vi "FaKI State Machine.vi"() -> ()   [LabVIEW 2023, in "FaKI State Machine.lvlib"]
doc: "The Producer-Consumer version of JKI State Machine.\n\nThis VI template must be instantiated by placing it on the block diagram of a new blank VI directly from the palettes. Do not use this template directly."
uses:
  FaKI State Machine.lvlib
  <vilib>/Utility/error.llb/Clear Errors.vi
panel:
  in  "Exit":bool
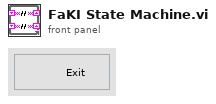
[diagram p1: front panel]
types:
  T1 = enum32{"Invalid", "Standard", "Closed", "Hidden", "Minimized", "Maximized"}
  T2 = enum32{"invalid app kind", "Development System", "Run Time System", "Student Edition", "Embedded LabVIEW", "Evaluation", "Custom"}
  T3 = cluster{"Core":cluster{"Current VI Reference":refnum<vi>, "Close Panel on Exit?":bool}, "Your Boolean data":bool, "Your string data":string}
  T4 = cluster{"Current VI Reference":refnum<vi>, "Close Panel on Exit?":bool}
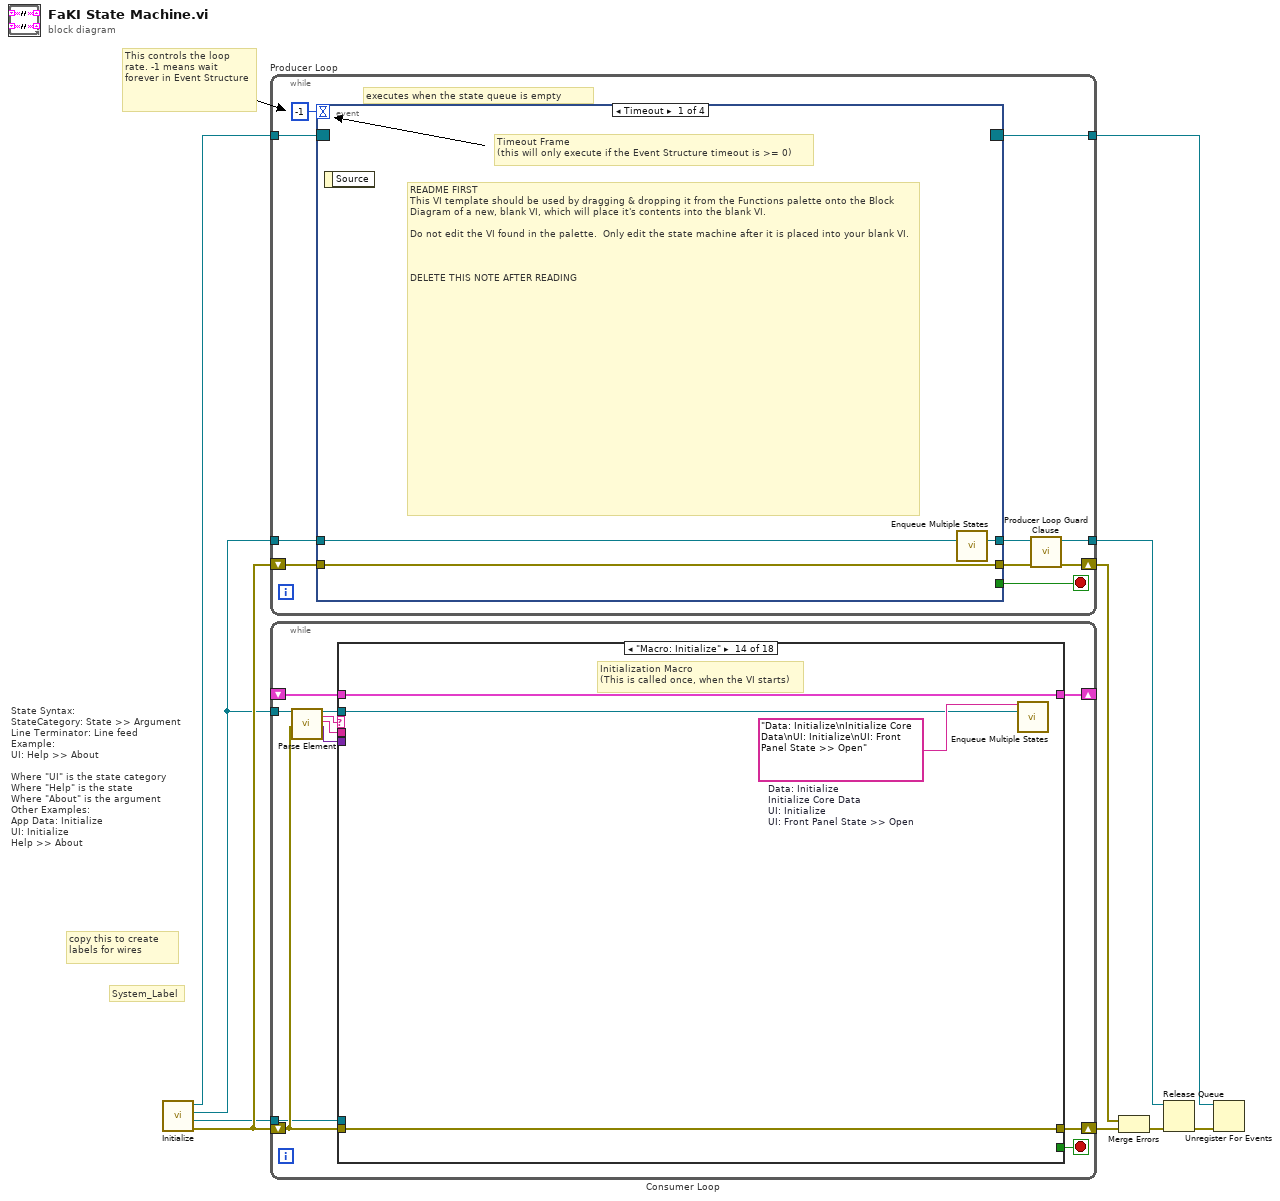
[diagram p0: block diagram]
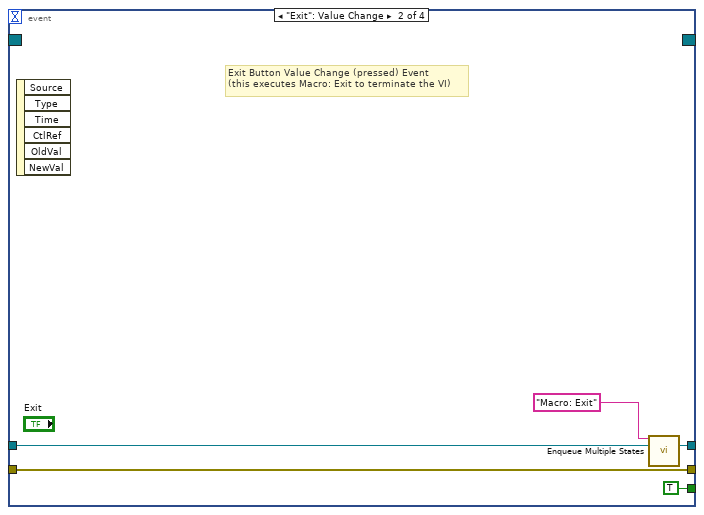
[diagram p2: hidden frame]
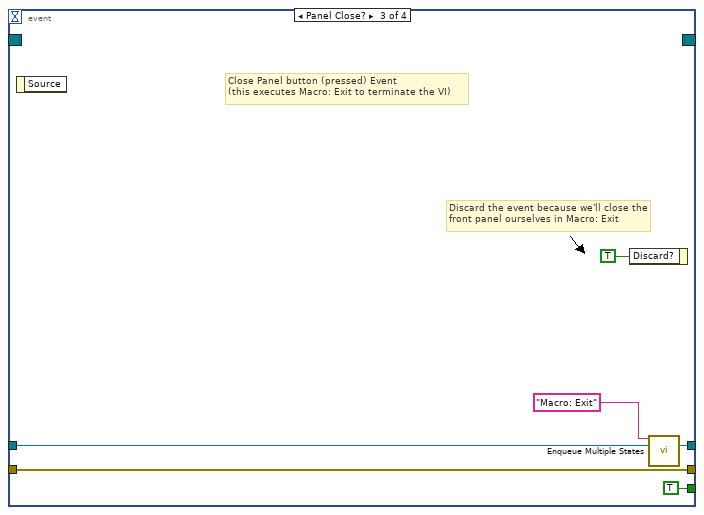
[diagram p3: hidden frame]
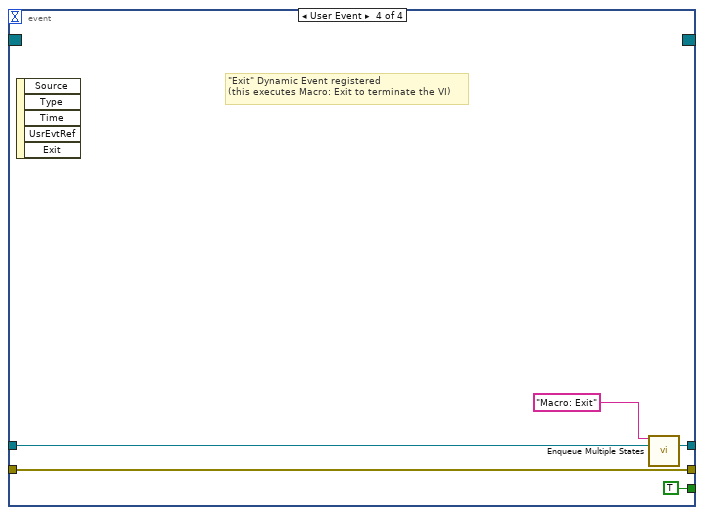
[diagram p4: hidden frame]
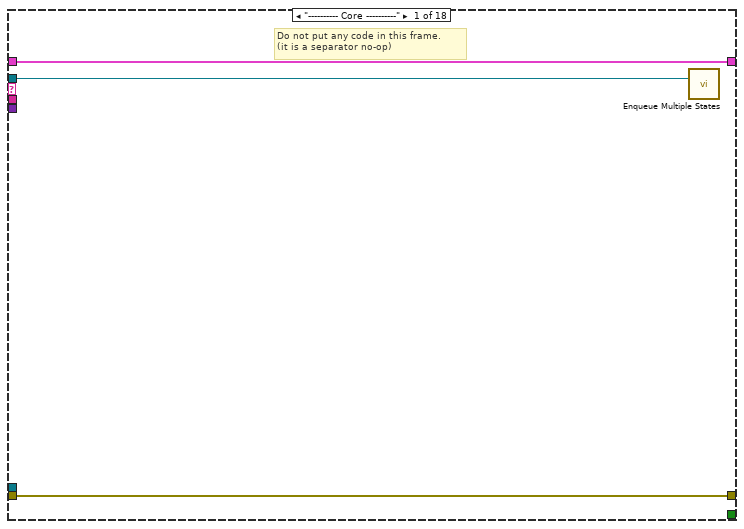
[diagram p5: hidden frame]
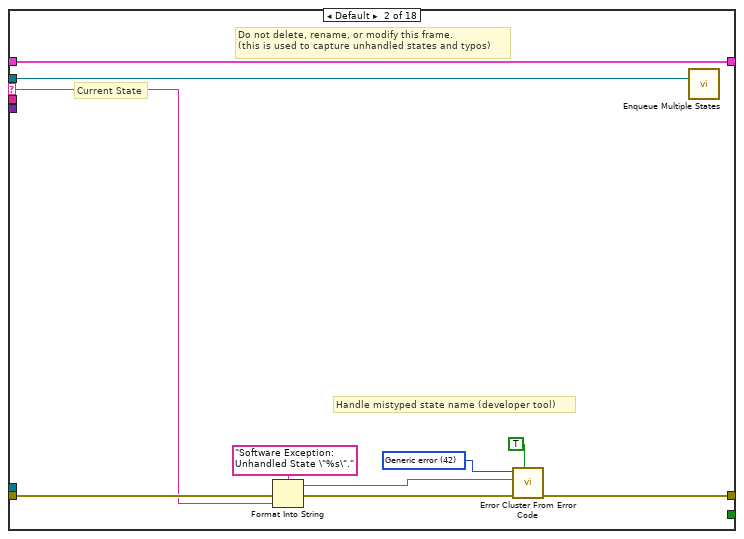
[diagram p6: hidden frame]
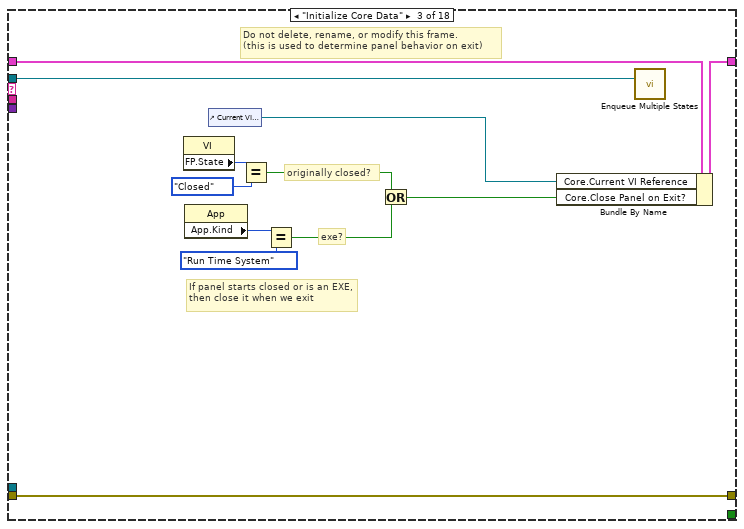
[diagram p7: hidden frame]
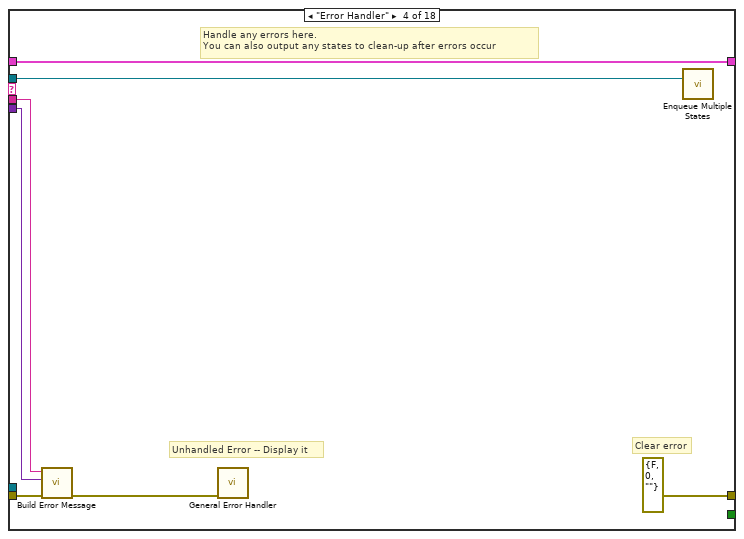
[diagram p8: hidden frame]
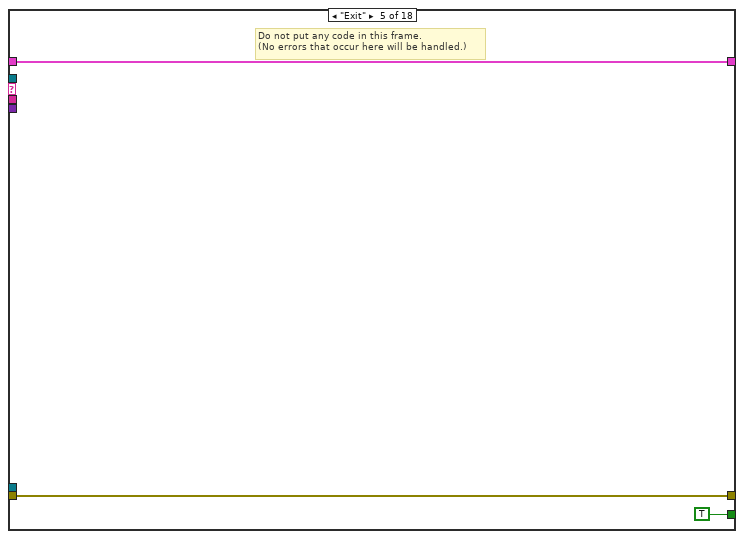
[diagram p9: hidden frame]
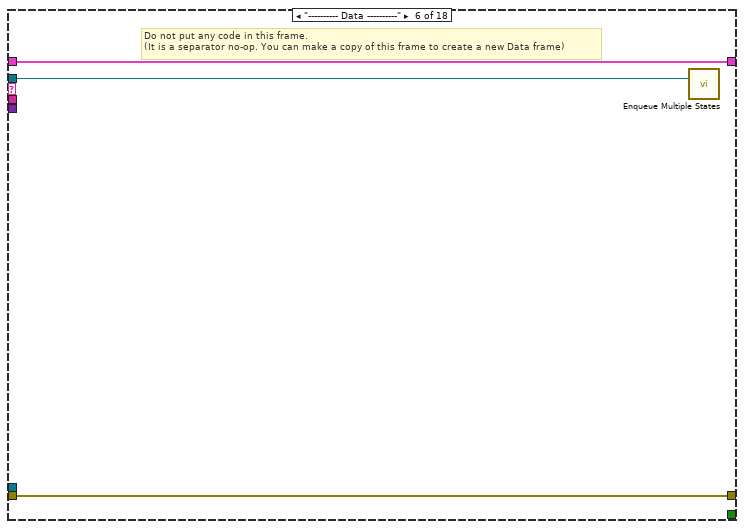
[diagram p10: hidden frame]
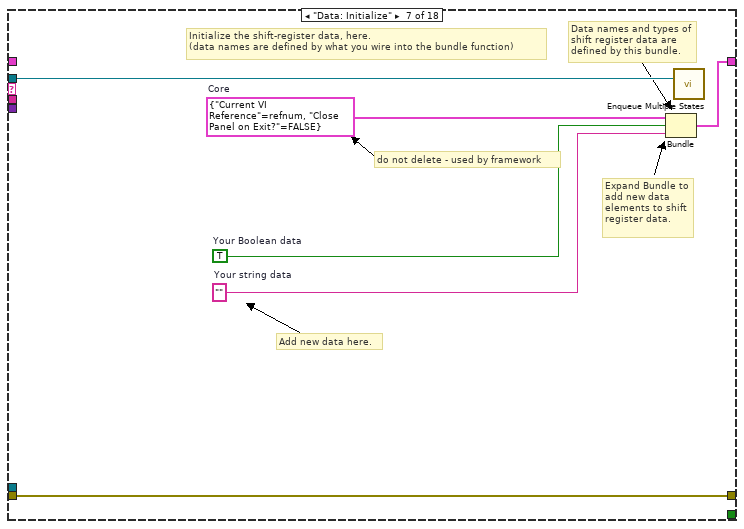
[diagram p11: hidden frame]
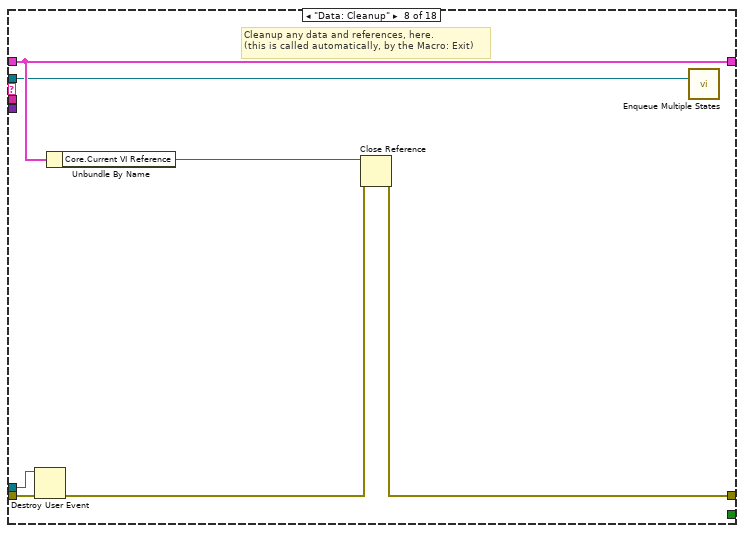
[diagram p12: hidden frame]
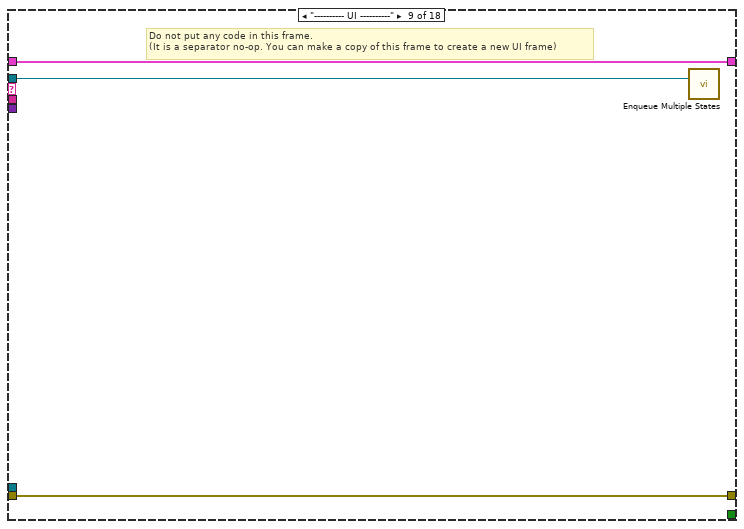
[diagram p13: hidden frame]
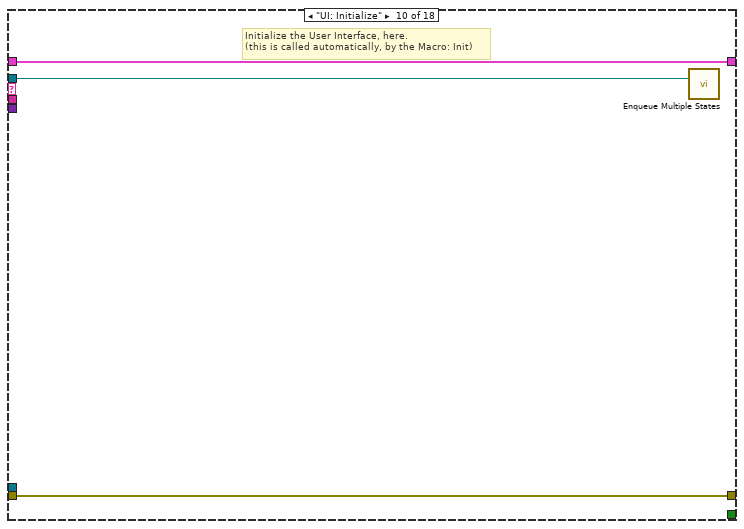
[diagram p14: hidden frame]
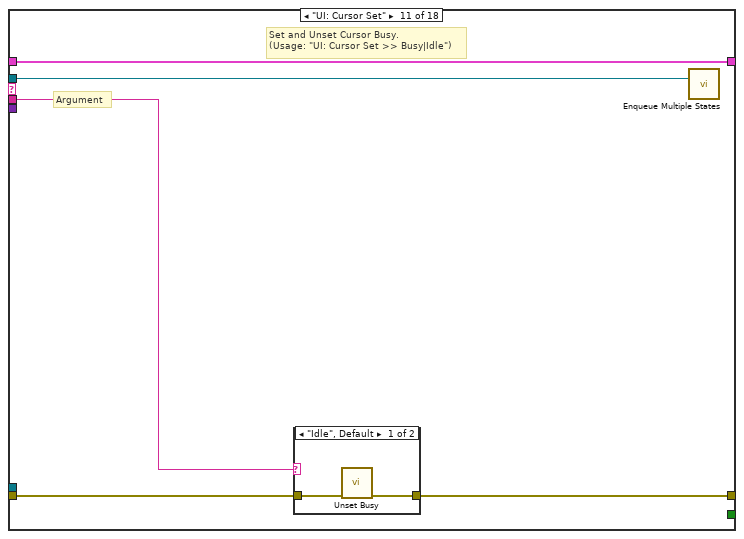
[diagram p15: hidden frame]
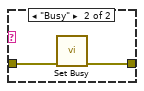
[diagram p16: hidden frame]
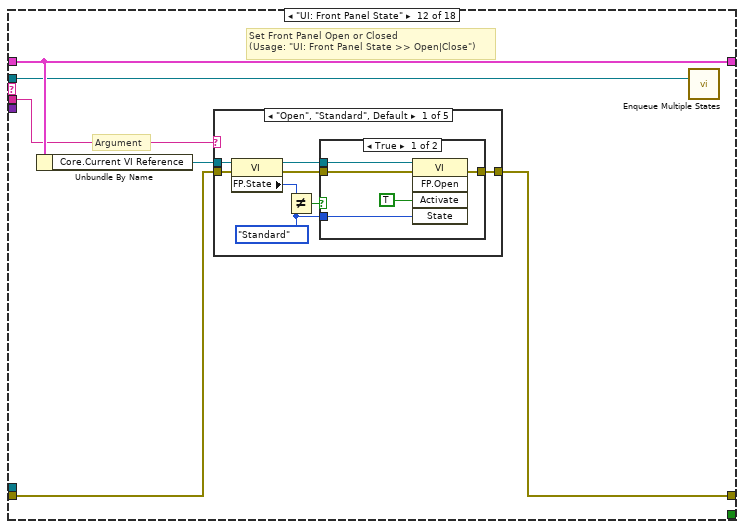
[diagram p17: hidden frame]
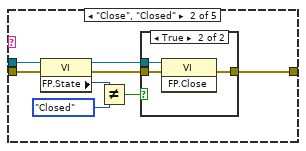
[diagram p19: hidden frame]
diagram:
  # "This controls the loop rate. -1 means wait forever in Event Structure"
  # "State Syntax:\nStateCategory: State >> Argument\nLine Terminator: Line feed\nExample:\nUI: Help >> About\n\nWhere \"UI\" is the state category\nWhere \"Help\" is the state\nWhere \"About\" is the argument\nOther Examples:\nApp Data: Initialize\nUI: Initialize\nHelp >> About"
  # "copy this to create labels for wires"
  # "System_Label"
  n1 = call "Initialize.vi"() -> ("error out"=w6:errorcluster, "Exit Event out"=w3:refnum<user-event>, "queue out"=w5:refnum<queue>, "Event Registration Refnum out"=w4:refnum<event-registration>)  [unwired: 8 in]
  n2 = while "Producer Loop" {
    shift-right: [w15] -> w9
    shift-left: w6 -> [w20]
    tunnel: w4 -> [w12]
    tunnel: w5 -> [w18]
    tunnel: [w13] -> w7
    tunnel: [w11] -> w1
    stop <- w17 stop-if-true
    # "executes when the state queue is empty"
    n3 = event shown="[0] Timeout" {
      selector: w12 -> [_ _ _ _]
      dyn-events: [_ _ _ _] -> w11
      timeout: -1 ("Timeout") -> [_ _ _ _]
      tunnel: [w21 w28 w34 w39] -> w16
      tunnel: w20 -> [w21 w28 w34 w39]
      tunnel: w18 -> [w22 w27 w31 w37]
      tunnel: [w23 w25 w30 w36] -> w14
      tunnel: [_ TRUE TRUE TRUE] -> w17
      event Timeout {
        # "README FIRST\nThis VI template should be used by dragging & dropping it from the Functions palette onto the Block Diagram of a new, blank VI, which will place it's contents into the blank VI.\n\nDo not edit the VI found in the palette.  Only edit the state machine after it is placed into your blank VI.\n\n\n\nDELETE THIS NOTE AFTER READING"
        # "Timeout Frame\n(this will only execute if the Event Structure timeout is >= 0)"
        n4 = event-data() -> ()  [unwired: 1 in, 1 out]
        n5 = call "Enqueue Multiple States.vi"("queue in"=w22) -> ("queue out"=w23:refnum<queue>)  [unwired: 14 in]
      }
      event "Exit": Value Change {
        # "Exit Button Value Change (pressed) Event\n(this executes Macro: Exit to terminate the VI)"
        n6 = event-data() -> ()  [unwired: 1 in, 6 out]
        n7 = call "Enqueue Multiple States.vi"("State(s) at Front"="Macro: Exit", "queue in"=w27) -> ("queue out"=w25:refnum<queue>)  [unwired: 13 in]
      }
      event Panel Close? {
        # "Discard the event because we'll close the front panel ourselves in Macro: Exit"
        # "Close Panel button (pressed) Event\n(this executes Macro: Exit to terminate the VI)"
        n8 = event-data() -> ()  [unwired: 1 in, 1 out]
        n9 = event-data("Discard?"=TRUE) -> ()  [unwired: 1 in, 1 out]
        n10 = call "Enqueue Multiple States.vi"("State(s) at Front"="Macro: Exit", "queue in"=w31) -> ("queue out"=w30:refnum<queue>)  [unwired: 13 in]
      }
      event User Event {
        # "\"Exit\" Dynamic Event registered\n(this executes Macro: Exit to terminate the VI)"
        n11 = event-data() -> ()  [unwired: 1 in, 5 out]
        n12 = call "Enqueue Multiple States.vi"("State(s) at Front"="Macro: Exit", "queue in"=w37) -> ("queue out"=w36:refnum<queue>)  [unwired: 13 in]
      }
    }
    n13 = call "Producer Loop Guard Clause.vi"("error in (no error)"=w16, "queue in"=w14) -> ("error out"=w15:errorcluster, "queue out"=w13:refnum<queue>)  [unwired: 8 in]
  }
  n14 = while "Consumer Loop" {
    shift-right: [w47] -> _
    shift-left: _ -> [w46]
    shift-right: [w50] -> w10
    shift-left: w6 -> [w49]
    tunnel: w5 -> [w45]
    tunnel: w3 -> [w40]
    stop <- w48 stop-if-true
    n15 = call "Parse Element.vi"("queue in"=w45, "error in (no error)"=w49) -> ("queue out"=w44:refnum<queue>, "State"=w43:string, "Arg"=w42:string, "Data"=w41:variant)  [unwired: 14 in]
    n16 = case shown="\"Macro: Initialize\"" w43 {
      selector: w43 -> [_ w55 _ _ _ _ _ _ _ _ _ _ _ _ _ _ _ _]
      tunnel: w44 -> [w51 w54 w64 w80 _ w86 w89 w98 w102 w105 w108 w117 w188 w191 w198 w204 w207 w210]
      tunnel: w42 -> [_ _ _ w76 _ _ _ _ _ _ w109 w118 _ _ _ _ _ _]
      tunnel: w46 -> [w52 w57 w70 w81 w84 w87 _ w99 w103 w106 w110 w120 w189 w193 w202 w205 w208 w211]
      tunnel: [w53 w62 w75 errorcluster {"status"=FALSE, "code"=0, "source"=""} ("error out") w85 w88 w94 w101 w104 w107 w111 w121 w190 w194 w203 w206 w209 w212] -> w50
      tunnel: w49 -> [w53 w61 w75 w79 w85 w88 w94 w97 w104 w107 w112 w122 w190 w194 w203 w206 w209 w212]
      tunnel: [_ _ _ _ TRUE _ _ _ _ _ _ _ _ _ _ _ _ _] -> w48
      tunnel: [w52 w57 w74 w81 w84 w87 w93 w99 w103 w106 w110 w120 w189 w193 w202 w205 w208 w211] -> w47
      tunnel: w41 -> [_ _ _ w77 _ _ _ _ _ _ _ _ _ _ _ _ _ _]
      tunnel: w40 -> [_ _ _ _ _ _ _ w96 _ _ _ _ _ _ _ _ _ _]
      frame "---------- Core ----------" {
        # "Do not put any code in this frame.\n(it is a separator no-op)"
        n17 = call "Enqueue Multiple States.vi"("queue in"=w51) -> ()  [unwired: 14 in, 1 out]
      }
      frame Default {
        w59 = 42 items=["No error", "Argument error", "Memory is full", "Out of zone", "End of file", "File already open", "Generic file I/O error", "File not found", "File permission error", "Disk is full", "Duplicate path", "Too many files open", "System feature not enabled", "Resource file not found", "Cannot add resource", "Resource not found", "Image not found", "Image memory error", "Pen does not exist", "Config type invalid", "Config token not found", "Config parse error", "Config memory error", "Bad external code format", "Bad external code offset", "External code not present", "Null window", "Destroy window error", "Null menu", "Print aborted", "Bad print record", "Print driver error", "Windows error during printing", "Memory error during printing", "Print dialog error", "Generic print error", "Invalid device refnum", "Device not found", "Device parameter error", "Device unit error", "Cannot open device", "Device call aborted", "Generic error", "Cancelled by user", "Object ID too low", "Object ID too high", "Object not in heap", "Unknown heap", "Unknown object (invalid DefProc)", "Unknown object (DefProc not in table)", "Message out of range", "Invalid (null) method", "Unknown message", "Manager call not supported", "Bad address", "Network operation in progress", "Network operation timed out", "Connection is busy", "Network attribute not supported", "Network error", "Address in use", "System out of memory", "Connection aborted", "Connection refused", "Not connected", "Already connected", "Connection closed", "Initialization error (interapplication manager)", "Bad occurrence", "Wait on unbound occurrence handler", "Occurrence queue overflow", "Datalog type conflict", "Unused", "Unrecognized type (interapplication manager)", "Memory corrupt", "Failed to make temporary DLL", "Old CIN version", "Drag socket not found", "Failed to load drop-object", "Failed to register OLE object", "Failed to release OLE object", "Format specifier type mismatch", "Unknown format specifier", "Too few format specifiers", "Too many format specifiers", "Scan failed", "Newer CIN version", "Error converting to variant", "Runtime menu error", "Password tampered", "Variant attribute not found", "Incompatible variant data type", "Event data is not available", "Event Store is not present", "Occurrence is not found", "Event Queue is not created", "Event info is not available", "Refnum passed is NULL", "Error retrieving Class GUID", "Error retrieving CoClass GUID", "Error retrieving TypeLib GUID.", "Bad built application magic bytes.", "Specific driver is different from the specific driver associated with the Logical Name.", "There is no session opened to the class driver.", "Max Error", "MAX - Error with config objects", "MAX - Error loading configuration", "MAX - Group not supported"]
        # "Current State"
        # "Do not delete, rename, or modify this frame.\n(this is used to capture unhandled states and typos)"
        # "Handle mistyped state name (developer tool)"
        n18 = Format Into String(format string="Software Exception: Unhandled State \"%s\"." ("message"), error in=w61, w55) -> (resulting string=w58:string, error out=w63:errorcluster)  [unwired: 1 in]
        n19 = call <vilib>:"Error Cluster From Error Code.vi"("show call chain? (False)"=TRUE, "error in (no error)"=w63, "error message (\"\")"=w58, "error code (0)"=w59) -> ("error out"=w62:errorcluster)  [unwired: 5 in]
        n20 = call "Enqueue Multiple States.vi"("queue in"=w54) -> ()  [unwired: 14 in, 1 out]
      }
      frame "Initialize Core Data" {
        # "Do not delete, rename, or modify this frame.\n(this is used to determine panel behavior on exit)"
        # "originally closed?"
        # "exe?"
        # "If panel starts closed or is an EXE, then close it when we exit"
        n21 = property class="VI"() -> ("FP.State"=w67:T1)  [unwired: 2 in, 2 out]
        n22 = property class="App"() -> ("App.Kind"=w73:T2)  [unwired: 2 in, 2 out]
        n23 = control-ref of="Current VI Reference"() -> (w68:refnum<vi>)
        n24 = Equal?(x=w67, y=T1."Closed" ("Front Panel Window:State")) -> (x = y?=w65:bool)
        n25 = Equal?(x=w73, y=T2."Run Time System" ("Application:Kind")) -> (x = y?=w71:bool)
        n26 = Or(x=w65, y=w71) -> (x .or. y?=w69:bool)
        n27 = Bundle By Name(cluster=w70, "Core.Current VI Reference"=w68, "Core.Close Panel on Exit?"=w69) -> (w74:T3)
        n28 = call "Enqueue Multiple States.vi"("queue in"=w64) -> ()  [unwired: 14 in, 1 out]
      }
      frame "Error Handler" {
        # "Unhandled Error -- Display it"
        # "Handle any errors here.\nYou can also output any states to clean-up after errors occur"
        # "Clear error"
        n29 = call "Build Error Message.vi"("error in (no error)"=w79, "Data"=w77, "Arg"=w76) -> ("error out"=w78:errorcluster)  [unwired: 8 in]
        n30 = call <vilib>:"General Error Handler.vi"("error in (no error)"=w78) -> ()  [unwired: 10 in, 5 out]
        n31 = call "Enqueue Multiple States.vi"("queue in"=w80) -> ()  [unwired: 14 in, 1 out]
      }
      frame "Exit" {
        # "Do not put any code in this frame.\n(No errors that occur here will be handled.)"
      }
      frame "---------- Data ----------" {
        # "Do not put any code in this frame.\n(It is a separator no-op. You can make a copy of this frame to create a new Data frame)"
        n32 = call "Enqueue Multiple States.vi"("queue in"=w86) -> ()  [unwired: 14 in, 1 out]
      }
      frame "Data: Initialize" {
        w90 = T4 {"Current VI Reference"=refnum, "Close Panel on Exit?"=FALSE}  # Core
        w92 = TRUE  # Your Boolean data
        w91 = ""  # Your string data
        # "do not delete - used by framework"
        # "Expand Bundle to add new data elements to shift register data."
        # "Add new data here."
        # "Data names and types of shift register data are defined by this bundle."
        # "Initialize the shift-register data, here.\n(data names are defined by what you wire into the bundle function)"
        n33 = Bundle("Core"=w90, "Your Boolean data"=w92, "Your string data"=w91) -> (w93:T3)  [unwired: 1 in]
        n34 = call "Enqueue Multiple States.vi"("queue in"=w89) -> ()  [unwired: 14 in, 1 out]
      }
      frame "Data: Cleanup" {
        # "Cleanup any data and references, here.\n(this is called automatically, by the Macro: Exit)"
        n35 = Destroy User Event(user event=w96, error in=w97) -> (error out=w95:errorcluster)
        n36 = Unbundle By Name(w99) -> ("Core.Current VI Reference"=w100:refnum<vi>)
        n37 = Close Reference(reference=w100, error in (no error)=w95) -> (error out=w101:errorcluster)
        n38 = call "Enqueue Multiple States.vi"("queue in"=w98) -> ()  [unwired: 14 in, 1 out]
      }
      frame "---------- UI ----------" {
        # "Do not put any code in this frame.\n(It is a separator no-op. You can make a copy of this frame to create a new UI frame)"
        n39 = call "Enqueue Multiple States.vi"("queue in"=w102) -> ()  [unwired: 14 in, 1 out]
      }
      frame "UI: Initialize" {
        # "Initialize the User Interface, here.\n(this is called automatically, by the Macro: Init)"
        n40 = call "Enqueue Multiple States.vi"("queue in"=w105) -> ()  [unwired: 14 in, 1 out]
      }
      frame "UI: Cursor Set" {
        # "Argument"
        # "Set and Unset Cursor Busy.\n(Usage: \"UI: Cursor Set >> Busy|Idle\")"
        n41 = case shown="\"Idle\", Default" w109 {
          tunnel: w112 -> [w114 w116]
          tunnel: [w113 w115] -> w111
          frame "Idle", Default {
            n42 = call <vilib>:"Unset Busy.vi"("error in (no error)"=w114) -> ("error out"=w113:errorcluster)  [unwired: 10 in]
          }
          frame "Busy" {
            n43 = call <vilib>:"Set Busy.vi"("error in (no error)"=w116) -> ("error out"=w115:errorcluster)  [unwired: 9 in, 1 out]
          }
        }
        n44 = call "Enqueue Multiple States.vi"("queue in"=w108) -> ()  [unwired: 14 in, 1 out]
      }
      frame "UI: Front Panel State" {
        # "Argument"
        # "Set Front Panel Open or Closed\n(Usage: \"UI: Front Panel State >> Open|Close\")"
        n45 = Unbundle By Name(w120) -> ("Core.Current VI Reference"=w119:refnum<vi>)
        n46 = case shown="\"Open\", \"Standard\", Default" w118 {
          tunnel: w122 -> [w129 w143 w155 w168 w181]
          tunnel: [w130 w144 w156 w169 w182] -> w121
          tunnel: w119 -> [w127 w141 w153 w166 w179]
          frame "Open", "Standard", Default {
            w123 = T1."Standard" ("State")
            n47 = property class="VI"(reference=w127, error in=w129) -> (reference out=w126:refnum<vi>, error out=w128:errorcluster, "FP.State"=w125:T1)
            n48 = Not Equal?(x=w125, y=w123) -> (x != y?=w124:bool)
            n49 = case shown="True" w124 {
              tunnel: [w135 w136] -> w130
              tunnel: w128 -> [w134 w136]
              tunnel: w126 -> [w132 _]
              tunnel: w123 -> [w131 _]
              frame True {
                n50 = invoke class="VI" method="FP.Open"(reference=w132, error in=w134, "Activate"=TRUE, "State"=w131) -> (error out=w135:errorcluster)  [unwired: 1 in, 4 out]
              }
              frame False {
              }
            }
          }
          frame "Close", "Closed" {
            n51 = property class="VI"(reference=w141, error in=w143) -> (reference out=w140:refnum<vi>, error out=w142:errorcluster, "FP.State"=w138:T1)
            n52 = Not Equal?(x=w138, y=T1."Closed" ("Front Panel Window:State")) -> (x != y?=w137:bool)
            n53 = case shown="True" w137 {
              tunnel: [w145 w148] -> w144
              tunnel: w142 -> [w145 w147]
              tunnel: w140 -> [_ w146]
              frame False {
              }
              frame True {
                n54 = invoke class="VI" method="FP.Close"(reference=w146, error in=w147) -> (error out=w148:errorcluster)  [unwired: 1 in, 2 out]
              }
            }
          }
          frame "Hidden", "Hide" {
            w149 = T1."Hidden" ("State")
            n55 = property class="VI"(reference=w153, error in=w155) -> (reference out=w152:refnum<vi>, error out=w154:errorcluster, "FP.State"=w151:T1)
            n56 = Not Equal?(x=w151, y=w149) -> (x != y?=w150:bool)
            n57 = case shown="True" w150 {
              tunnel: [w160 w161] -> w156
              tunnel: w154 -> [w159 w161]
              tunnel: w152 -> [w158 _]
              tunnel: w149 -> [w157 _]
              frame True {
                n58 = invoke class="VI" method="FP.Open"(reference=w158, error in=w159, "State"=w157) -> (error out=w160:errorcluster)  [unwired: 2 in, 4 out]
              }
              frame False {
              }
            }
          }
          frame "Minimize", "Minimized" {
            w162 = T1."Minimized" ("State")
            n59 = property class="VI"(reference=w166, error in=w168) -> (reference out=w165:refnum<vi>, error out=w167:errorcluster, "FP.State"=w164:T1)
            n60 = Not Equal?(x=w164, y=w162) -> (x != y?=w163:bool)
            n61 = case shown="True" w163 {
              tunnel: [w173 w174] -> w169
              tunnel: w167 -> [w172 w174]
              tunnel: w165 -> [w171 _]
              tunnel: w162 -> [w170 _]
              frame True {
                n62 = invoke class="VI" method="FP.Open"(reference=w171, error in=w172, "State"=w170) -> (error out=w173:errorcluster)  [unwired: 2 in, 4 out]
              }
              frame False {
              }
            }
          }
          frame "Maximize", "Maximized" {
            w175 = T1."Maximized" ("State")
            n63 = property class="VI"(reference=w179, error in=w181) -> (reference out=w178:refnum<vi>, error out=w180:errorcluster, "FP.State"=w177:T1)
            n64 = Not Equal?(x=w177, y=w175) -> (x != y?=w176:bool)
            n65 = case shown="True" w176 {
              tunnel: [w186 w187] -> w182
              tunnel: w180 -> [w185 w187]
              tunnel: w178 -> [w184 _]
              tunnel: w175 -> [w183 _]
              frame True {
                n66 = invoke class="VI" method="FP.Open"(reference=w184, error in=w185, "State"=w183) -> (error out=w186:errorcluster)  [unwired: 2 in, 4 out]
              }
              frame False {
              }
            }
          }
        }
        n67 = call "Enqueue Multiple States.vi"("queue in"=w117) -> ()  [unwired: 14 in, 1 out]
      }
      frame "---------- Macro ----------" {
        # "Do not put any code in this frame.\n(It is a separator no-op. You can make a copy of this frame to create a new Macro frame)"
        n68 = call "Enqueue Multiple States.vi"("queue in"=w188) -> ()  [unwired: 14 in, 1 out]
      }
      frame "Macro: Initialize" {
        w192 = "Data: Initialize\nInitialize Core Data\nUI: Initialize\nUI: Front Panel State >> Open"  # Data: Initialize Initialize Core Data UI: Initialize UI: Front Panel State >> Open
        # "Initialization Macro\n(This is called once, when the VI starts)"
        n69 = call "Enqueue Multiple States.vi"("State(s) at Front"=w192, "queue in"=w191) -> ()  [unwired: 13 in, 1 out]
      }
      frame "Macro: Exit" {
        # "Exit Macro\n(This is called once, when the VI exits)"
        n70 = Unbundle By Name(w202) -> ("Core.Close Panel on Exit?"=w201:bool)
        n71 = Select(t="UI: Front Panel State >> Close\n", s=w201, f="") -> (s? t:f=w197:string)
        n72 = Concatenate Strings(w197, "Data: Cleanup\nExit") -> (w195:string)
        n73 = call "Enqueue Multiple States.vi"("State(s) at Front"=w195, "queue in"=w198) -> ()  [unwired: 13 in, 1 out]
      }
      frame "---------- New Category ----------" {
        # "Template Separator\n(You can make a copy of, or modify, this frame)"
        n74 = call "Enqueue Multiple States.vi"("queue in"=w204) -> ()  [unwired: 14 in, 1 out]
      }
      frame "New Category: 1" {
        # "Your code here.\n(You can make a copy of, or modify, this frame)"
        n75 = call "Enqueue Multiple States.vi"("queue in"=w207) -> ()  [unwired: 14 in, 1 out]
      }
      frame "New Category: 2" {
        # "Your code here.\n(You can make a copy of, or modify, this frame)"
        n76 = call "Enqueue Multiple States.vi"("queue in"=w210) -> ()  [unwired: 14 in, 1 out]
      }
    }
  }
  n77 = Merge Errors(w9, w10) -> (w8:errorcluster)
  n78 = Release Queue(queue=w7, error in (no error)=w8) -> (error out=w2:errorcluster)  [unwired: 1 in, 2 out]
  n79 = Unregister For Events(event registration refnum=w1, error in=w2) -> ()  [unwired: 1 out]
